vi "SENSOR DAQ.vi"() -> ()   [LabVIEW 2018]
panel:
  out "Numeric":dbl
  in  "stop":bool
  out ".not. x?":bool
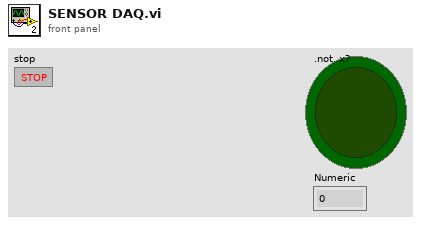
[diagram p1: front panel]
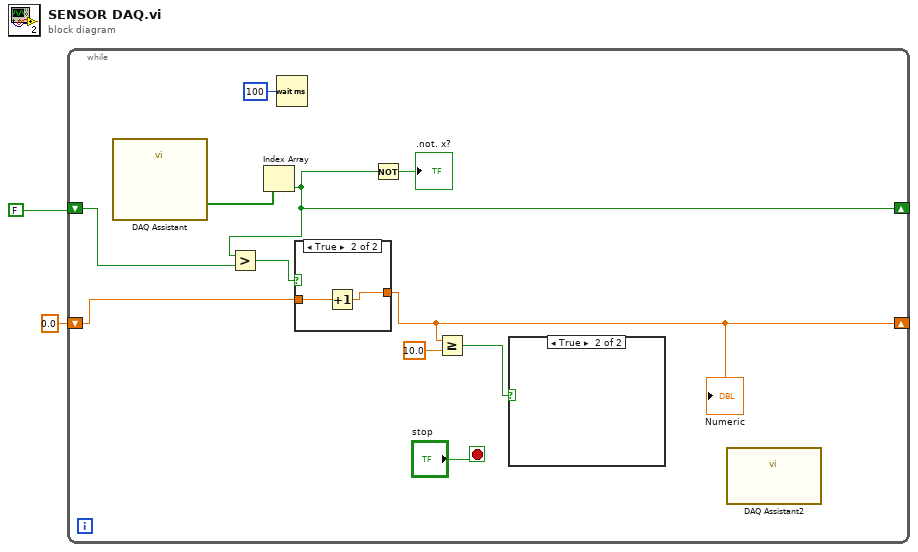
[diagram p0: block diagram]
diagram:
  n1 = while {
    shift-right: [w7] -> _
    shift-left: FALSE -> [w8]
    shift-right: [w5] -> _
    shift-left: 0.0 -> [w6]
    stop <- "stop" stop-if-true
    n2 = call "DAQ Assistant"() -> ("data"=w13:bool[])  [unwired: 17 in, 2 out]
    n3 = Index Array(array=w13) -> (element=w7:bool)  [unwired: 1 in]
    n4 = Greater?(x=w7, y=w8) -> (0:w9:bool)
    n5 = Wait (ms)(milliseconds to wait=u32 100) -> ()  [unwired: 1 out]
    n6 = case shown="True" w9 {
      tunnel: [w14 w16] -> w5
      tunnel: w6 -> [w14 w15]
      frame False {
      }
      frame True {
        n7 = Increment(x=w15) -> (x+1=w16:dbl)
      }
    }
    "Numeric" <- w5
    n8 = Not(x=w7) -> (.not. x?=→".not. x?":bool)
    n9 = Greater Or Equal?(x=w5, y=10.0) -> (x >= y?=w3:bool)
    n10 = case shown="True" w3 {
      frame False {
      }
      frame True {
      }
    }
    n11 = call "DAQ Assistant2"() -> ()  [unwired: 12 in]
  }
